vi "LabVIEW.ini File Path.vi"() -> (14 "appended path":path)   [LabVIEW 2017]
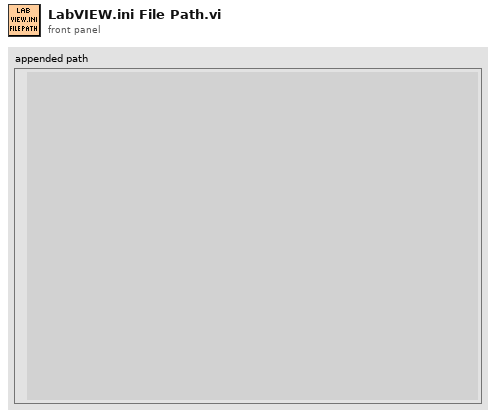
[diagram p1: front panel]
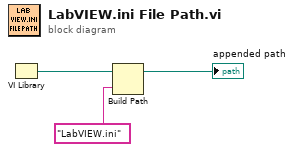
[diagram p0: block diagram]
diagram:
  n1 = VI Library() -> (path=w1:path)
  n2 = Build Path(base path=w1, name or relative path="LabVIEW.ini") -> (appended path=→"appended path":path)
